vi "Init 1.vi"(3 "Container State":T3 caption="Container-Status", 4 "Previous State":variant caption="Voriger Zustand", 5 "Previous Version":T2 caption="Vorherige Version") -> (2 "Current State":T1 caption="Aktueller Zustand")   [LabVIEW 2010, in "util.lvlib" / "XControl 1.xctl"]
uses:
  XControl 1.xctl
  Zustand 1.ctl
  <vilib>/_xctls/Container State.ctl
  <vilib>/_xctls/Version.ctl
  <vilib>/_xctls/XControlSupport.lvlib
panel:
  in  "Default Indicator State":T1 caption="Standard-Anzeigeelementzustand"
  in  "Default Control State":T1 caption="Standard-Bedienelementzustand"
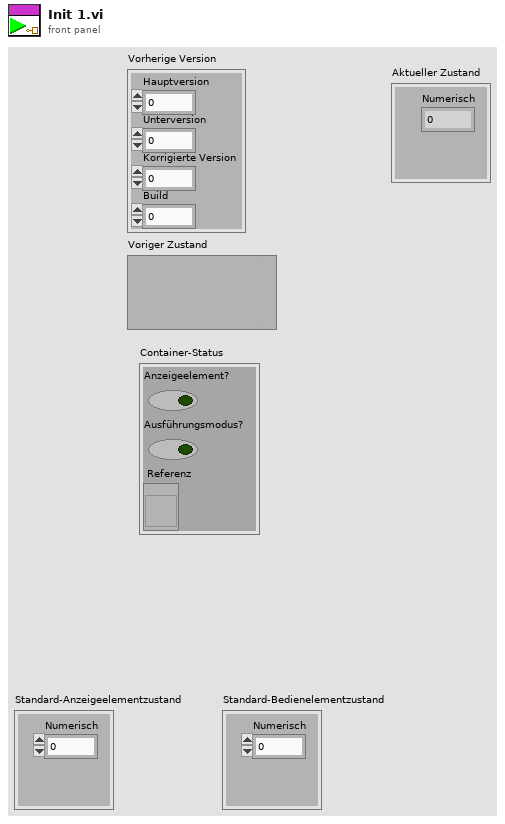
[diagram p1: front panel]
types:
  T1 = typedef "util.lvlib/XControl 1.xctl/Zustand 1.ctl" = cluster{"Numeric":dbl}
  T2 = typedef "XControlSupport.lvlib/Version.ctl" = cluster{"Major":u16, "Minor":u16, "Fix":u16, "Build":u16}
  T3 = typedef "XControlSupport.lvlib/Container State.ctl" = cluster{"Indicator?":bool, "Run Mode?":bool, " Refnum":refnum<vi>}
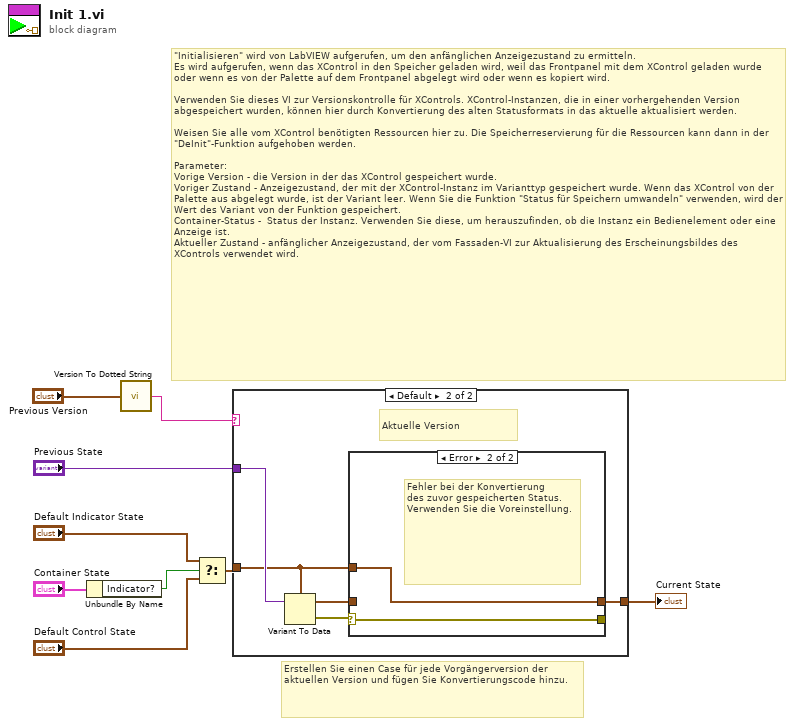
[diagram p0: block diagram]
diagram:
  # "Erstellen Sie einen Case für jede Vorgängerversion der aktuellen Version und fügen Sie Konvertierungscode hinzu."
  # "\"Initialisieren\" wird von LabVIEW aufgerufen, um den anfänglichen Anzeigezustand zu ermitteln.\nEs wird aufgerufen, wenn das XControl in den Speicher geladen wird, weil das Frontpanel mit dem XControl geladen wurde oder wenn es von der Palette auf dem Frontpanel abgelegt wird oder wenn es kopiert wird.\n\nVerwenden Sie dieses VI zur Versionskontrolle für XControls. XControl-Instanzen, die in einer vorhergehenden Version abgespeichert wurden, können hier durch Konvertierung des alten Statusformats in das aktuelle aktualisiert werden.\n\nWeisen Sie alle vom XControl benötigten Ressourcen hier zu. Die Speicherreservierung für die Ressourcen kann dann in der \"DeInit\"-Funktion aufgehoben werden.\n\nParameter:\nVorige Version - die Version in der das XControl gespeichert wurde.\nVoriger Zustand - Anzeigezustand, der mit der XControl-Instanz im Varianttyp gespeichert wurde. Wenn das XControl von der Palette aus abgelegt wurde, ist der Variant leer. Wenn Sie die Funktion \"Status für Speichern umwandeln\" verwenden, wird der Wert des Variant von der Funktion gespeichert. \nContainer-Status -  Status der Instanz. Verwenden Sie diese, um herauszufinden, ob die Instanz ein Bedienelement oder eine Anzeige ist.\nAktueller Zustand - anfänglicher Anzeigezustand, der vom Fassaden-VI zur Aktualisierung des Erscheinungsbildes des XControls verwendet wird."
  n1 = Unbundle By Name("Container State") -> ("Indicator?"=w4:bool)
  n2 = call <vilib>:"Version To Dotted String.vi"("Version"="Previous Version") -> ("String Version"=w1:string)
  n3 = Select(t="Default Indicator State", s=w4, f="Default Control State") -> (s? t:f=w3:T1)
  n4 = case shown="Default" w1 {
    tunnel: "Previous State" -> [_ w15]
    tunnel: [w10 w11] -> w8
    tunnel: w3 -> [w10 w12]
    frame "0.0.0.0" {
      # "Gerade erstellt, verwende Standardzustand"
    }
    frame Default {
      # "Aktuelle Version"
      n5 = Variant To Data(Variant=w15, type=w12) -> (error out=w14:errorcluster, data=w13:T1)  [unwired: 1 in]
      n6 = case shown="Error" w14 {
        selector: w14 -> [w17 w18]
        tunnel: w13 -> [w16 _]
        tunnel: [w16 w19] -> w11
        tunnel: w12 -> [_ w19]
        tunnel: [w17 w18] -> _
        frame No Error {
        }
        frame Error {
          # "Fehler bei der Konvertierung \ndes zuvor gespeicherten Status. Verwenden Sie die Voreinstellung."
        }
      }
    }
  }
  "Current State" <- w8
